vi "Configure Reference Mass.vi"(8 "error in (no error)":errorcluster, 10 "Reference Mass [g]":dbl=1.0, 11 "VISA resource name":refnum<visa-resource-name>) -> (0 "error out":errorcluster, 3 "VISA resource name out":refnum<visa-resource-name>)   [LabVIEW 2017, in "RadWag balances and scales.lvlib"]
doc: "Sets the reference mass value in deviations mode.\nThis VI works properly when balance works in deviations mode. (To configure work mode use Utility -> Set work mode)"
uses:
  <instrlib>/Prev/RadWag Continuous Read Folder/RadWag balances and scales.lvlib
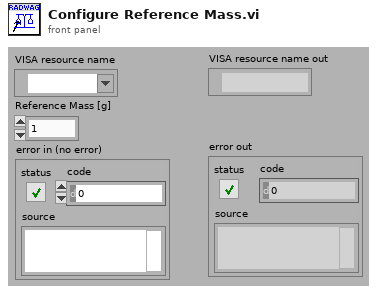
[diagram p1: front panel]
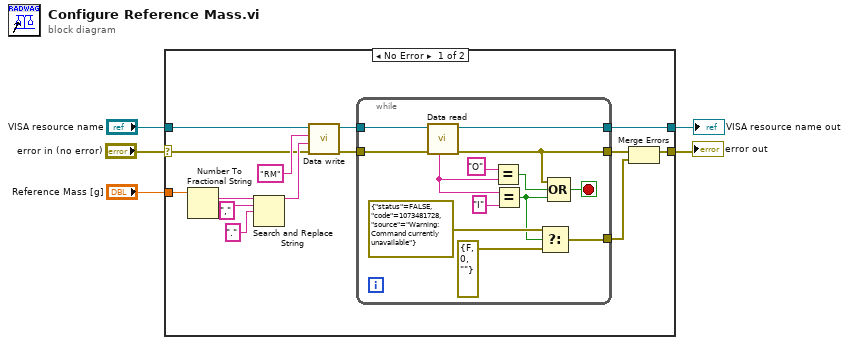
[diagram p0: block diagram]
diagram:
  n1 = case shown="No Error" "error in (no error)" {
    selector: "error in (no error)" -> [w9 w33]
    tunnel: "VISA resource name" -> [w19 w34]
    tunnel: [w16 w34] -> w4
    tunnel: [w7 w33] -> w3
    tunnel: "Reference Mass [g]" -> [w14 _]
    frame No Error {
      n2 = Number To Fractional String(number=w14) -> (F-format string=w13:string)  [unwired: 3 in]
      n3 = Search and Replace String(input string=w13, search string=",", replace string="." ("replace string (\"\")")) -> (result string=w10:string)  [unwired: 5 in, 3 out]
      n4 = call <instrlib>:"Data write.vi"("error in (no error)"=w9, "Parameter"=w10, "ID"="RM", "VISA resource name"=w19) -> ("error out"=w17:errorcluster, "VISA resource name out"=w18:refnum<visa-resource-name>)  [unwired: 6 in]
      n5 = while {
        tunnel: w18 -> [w32]
        tunnel: w17 -> [w31]
        tunnel: [w30] -> w16
        tunnel: [w25] -> w8
        tunnel: [w20] -> w6
        stop <- w26 stop-if-true
        n6 = call <instrlib>:"Data read.vi"("error in (no error)"=w31, "VISA resource name"=w32) -> ("error out"=w25:errorcluster, "VISA resource name out"=w30:refnum<visa-resource-name>, "Status"=w29:string)  [unwired: 3 in, 4 out]
        n7 = Equal?(x="O", y=w29) -> (x = y?=w24:bool)
        n8 = Equal?(x=w29, y="I") -> (x = y?=w21:bool)
        n9 = Select(t=errorcluster {"status"=FALSE, "code"=1073481728, "source"="Warning: Command currently unavailable"}, s=w21, f=errorcluster {"status"=FALSE, "code"=0, "source"=""} ("error constant")) -> (s? t:f=w20:errorcluster)
        n10 = Compound Arithmetic op=OR(w25, w24, w21) -> (w26:bool)
      }
      n11 = Merge Errors(w8, w6) -> (w7:errorcluster)
    }
    frame Error {
    }
  }
  "VISA resource name out" <- w4
  "error out" <- w3
